vi "Write selected motor.vi"(8 "error in (no error)":errorcluster, 10 "Motor.lvclass":refnum<class "Motor.lvclass">, 11 "ICS in":refnum<class "ICS.lvclass">) -> (0 "error out":errorcluster, 3 "ICS out":refnum<class "ICS.lvclass">)   [LabVIEW 2018, in "ICS.lvclass"]
uses:
  ICS.lvclass
  Motor/Motor.lvclass
  ICS.lvclass/ICS.ctl
  MotorManager/MotorManager.lvclass
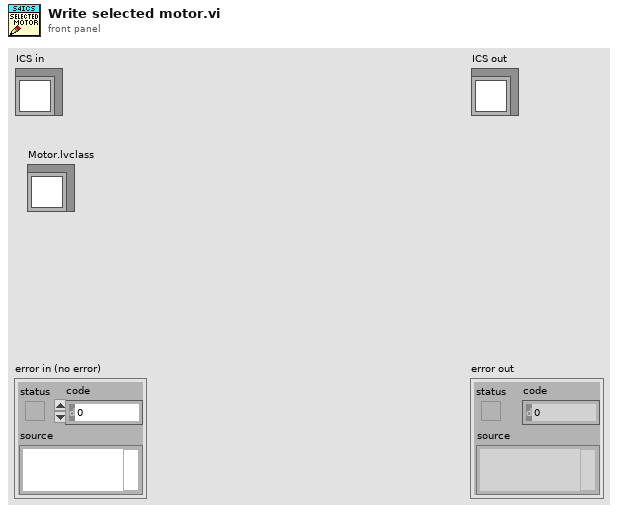
[diagram p1: front panel]
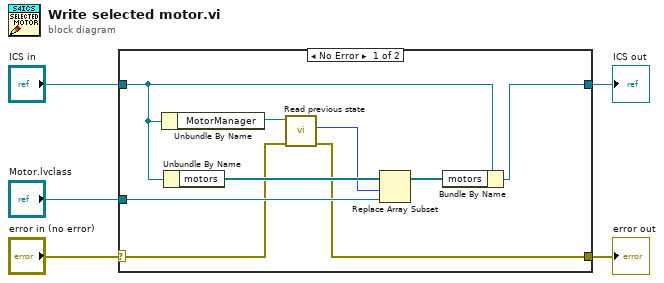
[diagram p0: block diagram]
diagram:
  n1 = case shown="No Error" "error in (no error)" {
    selector: "error in (no error)" -> [w10 w15]
    tunnel: [w9 w15] -> w4
    tunnel: [w14 w16] -> w2
    tunnel: "ICS in" -> [w7 w16]
    tunnel: "Motor.lvclass" -> [w11 _]
    frame No Error {
      n2 = Unbundle By Name(w7) -> ("MotorManager"=w6:refnum<class "MotorManager.lvclass">)
      n3 = Unbundle By Name(w7) -> ("motors"=w13:refnum<class "Motor.lvclass">[])
      n4 = call-dynamic "Read previous state.vi"("error in (no error)"=w10, "StateManager in"=w6) -> ("error out"=w9:errorcluster, "previousState"=w8:u32)  [unwired: 7 in, 1 out]
      n5 = Replace Array Subset(array=w13, new element=w11, index=w8) -> (w12:refnum<class "Motor.lvclass">[])
      n6 = Bundle By Name(cluster=w7, "motors"=w12) -> (w14:refnum<class "ICS.lvclass">)
    }
    frame Error {
    }
  }
  "error out" <- w4
  "ICS out" <- w2
